vi "SetMessageError.vi"(10 "error":errorcluster, 11 "message in":T1) -> (3 "message out":T1)   [LabVIEW 2017]
uses:
  <vilib>/addons/InsightCM/MessageBus/Base/controls/Message.ctl
  <vilib>/addons/InsightCM/MessageBus/Base/controls/MessageHeader.ctl
  <vilib>/addons/InsightCM/MessageBus/Base/controls/KeyValuePair.ctl
  <vilib>/addons/InsightCM/Utilities/PropertyHelpers/PropertyHelpers.lvlib
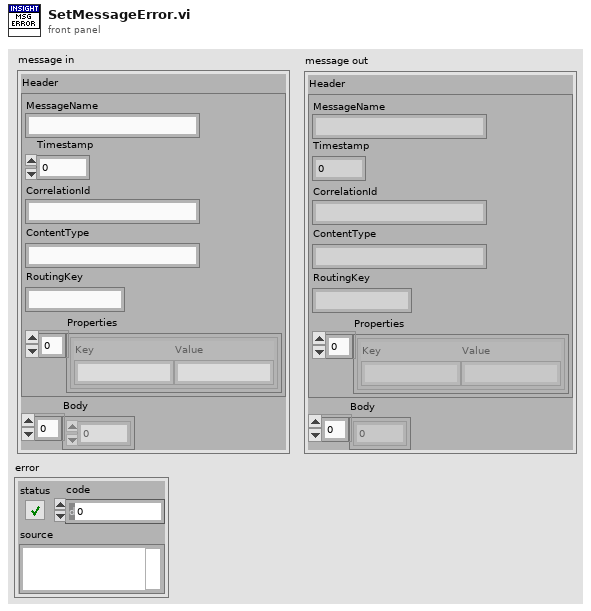
[diagram p1: front panel]
types:
  T1 = typedef "Message.ctl" = cluster{"Header":T2, "Body":u8[]}
  T2 = typedef "MessageHeader.ctl" = cluster{"MessageName":string, "Timestamp":i64, "CorrelationId":string, "ContentType":string, "RoutingKey":string, "Properties":T3[]}
  T3 = typedef "KeyValuePair.ctl" = cluster{"Key":string, "Value":string}
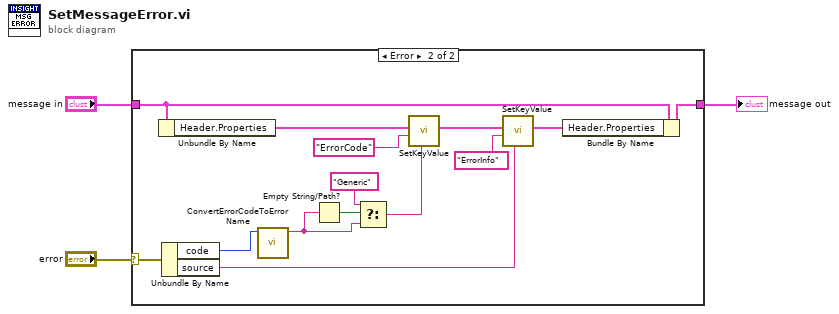
[diagram p0: block diagram]
diagram:
  n1 = case shown="Error" "error" {
    selector: "error" -> [_ w15]
    tunnel: "message in" -> [w4 w13]
    tunnel: [w4 w12] -> w2
    frame No Error {
    }
    frame Error {
      n2 = Unbundle By Name(w13) -> ("Header.Properties"=w11:T3[])
      n3 = Unbundle By Name(w15) -> ("code"=w14:i32, "source"=w8:string)
      n4 = call <vilib>:"ConvertErrorCodeToErrorName.vi"("ErrorCode"=w14) -> ("ErrorName"=w17:string)  [unwired: 9 in, 1 out]
      n5 = Empty String/Path?(string/path=w17) -> (empty?=w18:bool)
      n6 = Select(t="Generic" ("Key"), s=w18, f=w17) -> (s? t:f=w5:string)
      n7 = call <vilib>:"SetKeyValue.vi"("value"=w5, "key"="ErrorCode" ("Key"), "key value pairs"=w11) -> ("key value pairs out"=w10:T3[])  [unwired: 8 in]
      n8 = call <vilib>:"SetKeyValue.vi"("value"=w8, "key"="ErrorInfo" ("Key"), "key value pairs"=w10) -> ("key value pairs out"=w9:T3[])  [unwired: 8 in]
      n9 = Bundle By Name(cluster=w13, "Header.Properties"=w9) -> (w12:T1)
    }
  }
  "message out" <- w2
